vi "AMS5812_Convert Raw Pressure Temp.vi"(10 "Read Data":u8[](array[numeric])) -> (0 "Pressure rounded (mmHg)":dbl format="%.2f", 1 "Pressure (mmHg)":dbl format="%.2f", 2 "Pressure (mbar)":dbl format="%.2f", 3 "Pressure (Pa)":dbl, 4 "Temp (C)":dbl, 5 "Pressure (PSI)":dbl)   [LabVIEW 2020]
panel:
  out "LSB Temp":u8
  out "MSB Temp":u8
  out "LSB Pressure":u8
  out "MSB Pressure":u8
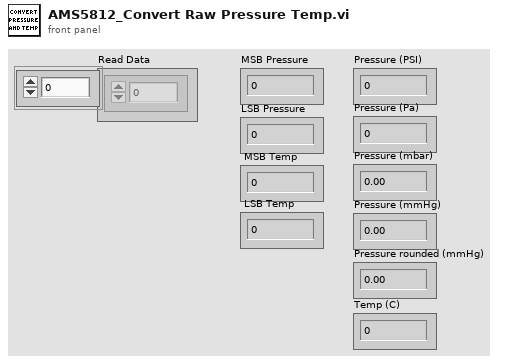
[diagram p1: front panel]
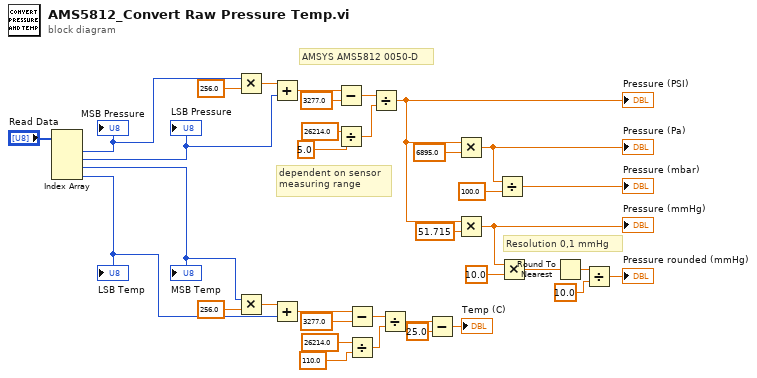
[diagram p0: block diagram]
diagram:
  # "Resolution 0,1 mmHg"
  # "dependent on sensor\nmeasuring range"
  # "AMSYS AMS5812 0050-D"
  n1 = Index Array(array="Read Data") -> (element #1=w35:u8, element #2=w33:u8, element #3=w15:u8, element #4=w14:u8)  [unwired: 4 in]
  "MSB Pressure" <- w35
  "LSB Pressure" <- w33
  "MSB Temp" <- w15
  "LSB Temp" <- w14
  n2 = Multiply(x=w35, y=256.0) -> (x*y=w34:dbl)
  n3 = Multiply(x=w15, y=256.0) -> (x*y=w20:dbl)
  n4 = Add(x=w34, y=w33) -> (x+y=w32:dbl)
  n5 = Add(x=w20, y=w14) -> (x+y=w21:dbl)
  n6 = Subtract(x=w32, y=3277.0) -> (x-y=w30:dbl)
  n7 = Divide(x=26214.0, y=5.0) -> (x/y=w29:dbl)
  n8 = Subtract(x=w21, y=3277.0) -> (x-y=w23:dbl)
  n9 = Divide(x=26214.0, y=110.0) -> (x/y=w24:dbl)
  n10 = Divide(x=w30, y=w29) -> (x/y=w8:dbl)
  "Pressure (PSI)" <- w8
  n11 = Divide(x=w23, y=w24) -> (x/y=w18:dbl)
  n12 = Subtract(x=w18, y=25.0) -> (x-y=→"Temp (C)":dbl)
  n13 = Multiply(x=w8, y=6895.0) -> (x*y=w12:dbl)
  "Pressure (Pa)" <- w12
  n14 = Multiply(x=w8, y=51.715) -> (x*y=w6:dbl)
  "Pressure (mmHg)" <- w6
  n15 = Divide(x=w12, y=100.0) -> (x/y=→"Pressure (mbar)":dbl)
  n16 = Multiply(x=w6, y=10.0) -> (x*y=w1:dbl)
  n17 = Round To Nearest(number=w1) -> (nearest integer value=w3:dbl)
  n18 = Divide(x=w3, y=10.0) -> (x/y=→"Pressure rounded (mmHg)":dbl)
